vi "Identify peaks.vi"(8 "error in (no error)":errorcluster, 10 "Parameters":T1={"Start frequency"=500000.0, "End frequency"=2000000.0, "Number of points"=38000, "Amplitude"=2.1, "Work folder"=path "C:/Data/RUS"} {"Amplitude" format="%#_6p"; "End frequency" format="%#_6p"; "Start frequency" format="%#_6p"}, 11 "RUS Measurement in":refnum<class "RUS Measurement.lvclass">) -> (0 "error out":errorcluster, 3 "RUS Measurement out":refnum<class "RUS Measurement.lvclass">)   [LabVIEW 2014, in "RUS Measurement.lvclass"]
uses:
  RUS Measurement.lvclass
  RUS Parameters.ctl
  RUS Measurement.lvclass/RUS Measurement.ctl
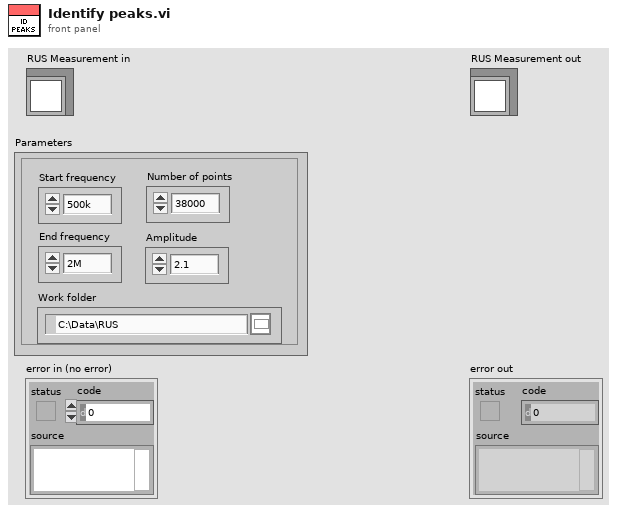
[diagram p1: front panel]
types:
  T1 = typedef "RUS Parameters.ctl" = cluster{"Start frequency":dbl, "End frequency":dbl, "Number of points":i32, "Amplitude":dbl, "Work folder":path}
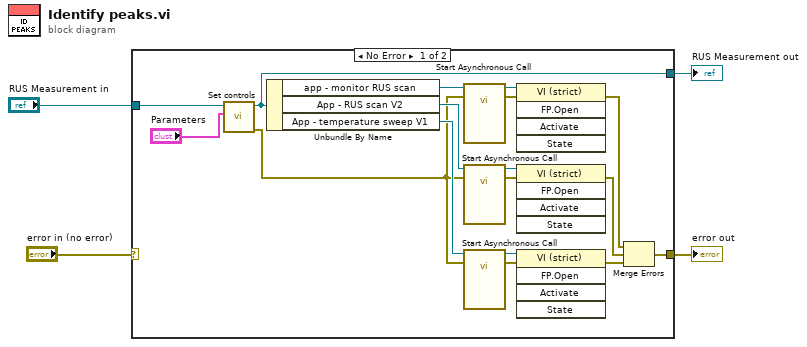
[diagram p0: block diagram]
diagram:
  n1 = case shown="No Error" "error in (no error)" {
    selector: "error in (no error)" -> [_ w23]
    tunnel: [w6 w23] -> w3
    tunnel: [w5 w22] -> w1
    tunnel: "RUS Measurement in" -> [w14 w22]
    frame No Error {
      n2 = call "Set controls.vi"("Parameters"="Parameters", "RUS Measurement in"=w14) -> ("error out"=w7:errorcluster, "RUS Measurement out"=w5:refnum<class "RUS Measurement.lvclass">)  [unwired: 8 in]
      n3 = Unbundle By Name(w5) -> ("app - monitor RUS scan"=w21:refnum<vi>, "App - RUS scan V2"=w16:refnum<vi>, "App - temperature sweep V1"=w11:refnum<vi>)
      n4 = call-by-ref "Start Asynchronous Call"(reference=w21, error in=w7) -> (reference out=w20:refnum<vi>, error out=w19:errorcluster)  [unwired: 12 in]
      n5 = call-by-ref "Start Asynchronous Call"(reference=w16, error in=w7) -> (reference out=w17:refnum<vi>, error out=w18:errorcluster)  [unwired: 14 in, 2 out]
      n6 = call-by-ref "Start Asynchronous Call"(reference=w11, error in=w7) -> (reference out=w10:refnum<vi>, error out=w9:errorcluster)  [unwired: 16 in]
      n7 = invoke class="VI (strict)" method="FP.Open"(reference=w20, error in=w19) -> (error out=w13:errorcluster)  [unwired: 3 in, 4 out]
      n8 = invoke class="VI (strict)" method="FP.Open"(reference=w17, error in=w18) -> (error out=w15:errorcluster)  [unwired: 3 in, 4 out]
      n9 = invoke class="VI (strict)" method="FP.Open"(reference=w10, error in=w9) -> (error out=w8:errorcluster)  [unwired: 3 in, 4 out]
      n10 = Merge Errors(w13, w15, w8) -> (w6:errorcluster)
    }
    frame Error {
    }
  }
  "error out" <- w3
  "RUS Measurement out" <- w1
